vi "Send.vi"() -> ()   [LabVIEW 2020]
panel:
  in  "Tab Control":enum32{"Data", "Error"}(tab)
  in  "Thermometer":dbl(slide) scale=0.0..100.0
  in  "stop":bool
  in  "PORT":i16=8081
  out "Bytes Written":i32
  out "error out":errorcluster
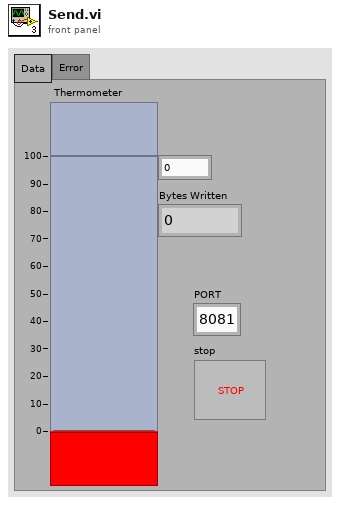
[diagram p1: front panel]
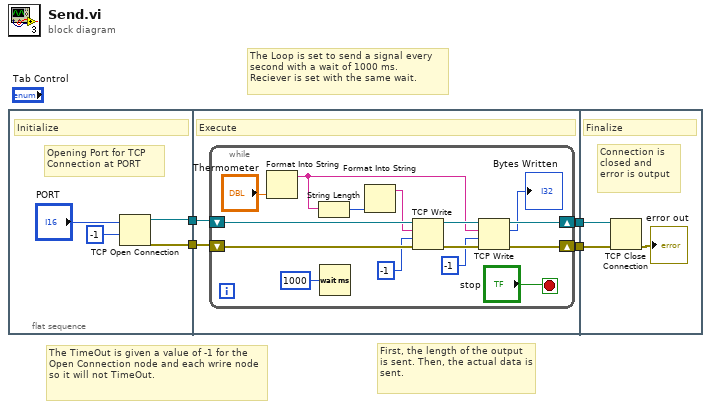
[diagram p0: block diagram]
diagram:
  # "The Loop is set to send a signal every \nsecond with a wait of 1000 ms.\nReciever is set with the same wait."
  # "First, the length of the output is sent. Then, the actual data is sent."
  # "The TimeOut is given a value of -1 for the Open Connection node and each wrire node so it will not TimeOut."
  n1 = flat-sequence {
    tunnel: [w5] -> w2
    tunnel: [w6] -> w1
    tunnel: [w11] -> w4
    tunnel: [w9] -> w3
    tunnel: w2 -> [w12]
    tunnel: w1 -> [w10]
    tunnel: w4 -> [w29]
    tunnel: w3 -> [w30]
    frame #0 {
      # "Opening Port for TCP \nConnection at PORT"
      # "Initialize"
      n2 = TCP Open Connection(remote port or service name="PORT", timeout ms (60000)=-1) -> (connection ID=w5:refnum<k5>, error out=w6:errorcluster)  [unwired: 3 in]
    }
    frame #1 {
      # "Execute"
      n3 = while {
        shift-right: [w25] -> w11
        shift-left: w12 -> [w27]
        shift-right: [w22] -> w9
        shift-left: w10 -> [w24]
        stop <- "stop" stop-if-true
        n4 = Format Into String("Thermometer") -> (resulting string=w15:string)  [unwired: 3 in, 1 out]
        n5 = String Length(string=w15) -> (length=w14:i32)
        n6 = Wait (ms)(milliseconds to wait=u32 1000) -> ()  [unwired: 1 out]
        n7 = Format Into String(w14) -> (resulting string=w13:string)  [unwired: 3 in, 1 out]
        n8 = TCP Write(connection ID=w27, data in=w13, error in (no error)=w24, 9:-1 ("timeout ms (25000)")) -> (connection ID out=w26:refnum<k5>, error out=w23:errorcluster)  [unwired: 1 out]
        n9 = TCP Write(connection ID=w26, data in=w15, error in (no error)=w23, 9:-1 ("timeout ms (25000)")) -> (connection ID out=w25:refnum<k5>, bytes written=→"Bytes Written":i32, error out=w22:errorcluster)
      }
    }
    frame #2 {
      # "Connection is closed and error is output"
      # "Finalize"
      n10 = TCP Close Connection(connection ID=w29, error in (no error)=w30) -> (error out=→"error out":errorcluster)  [unwired: 1 in, 1 out]
    }
  }
